vi "Execution Time.vi"() -> ()   [LabVIEW 2011]
panel:
  out "Resultant Array":dbl[](array[numeric])
  in  "stop":bool
  out "Execution Time":u32
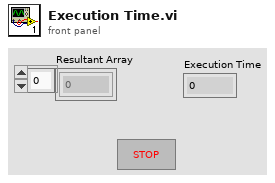
[diagram p1: front panel]
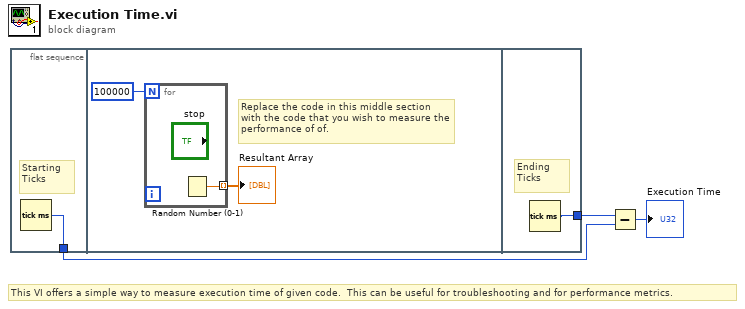
[diagram p0: block diagram]
diagram:
  # "This VI offers a simple way to measure execution time of given code.  This can be useful for troubleshooting and for performance metrics."
  n1 = flat-sequence {
    tunnel: [w4] -> w2
    tunnel: [w8] -> w3
    frame #0 {
      # "Starting Ticks"
      n2 = Tick Count (ms)() -> (millisecond timer value=w4:u32)
    }
    frame #1 {
      # "Replace the code in this middle section with the code that you wish to measure the performance of of."
      n3 = for {
        N: 100000 -> [_]
        tunnel: [w7] -> w5 mode=indexing
        n4 = Random Number (0-1)() -> (number: 0 to 1=w7:dbl)
      }
      "Resultant Array" <- w5
    }
    frame #2 {
      # "Ending Ticks"
      n5 = Tick Count (ms)() -> (millisecond timer value=w8:u32)
    }
  }
  n6 = Subtract(x=w3, y=w2) -> (x-y=→"Execution Time":u32)
